vi "Plot_Channels.vi"() -> (5 "Plug in titles":string[](array[string]), 7 "Plug in values":string[](array[string]))   [LabVIEW 2011]
uses:
  Globals/Meas_global.vi
panel:
  out "Stats out":T1
  out "Size 2":i32
  out "Size 1":i32
  out "Size 0":i32
  in  "interp. method":i32(ring) items=["nearest", "linear", "spline", "cubic Hermite", "Lagrange"]
  in  "index 2":i32=3
  out "XY Graph":cluster{"Time (ms)":dbl[], "Eng Values":dbl[]}[](graph)
  in  "index 1":i32=1
  in  "index 0":i32
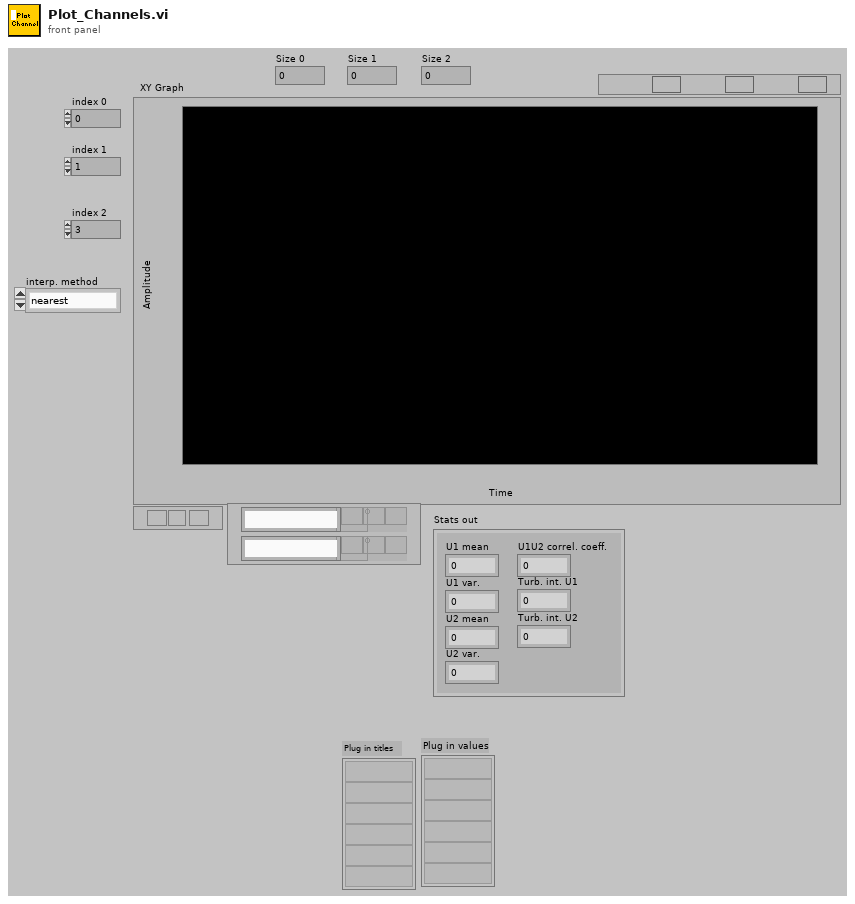
[diagram p1: front panel]
types:
  T1 = cluster{"U1 mean":dbl, "U1 var.":dbl, "U2 mean":dbl, "U2 var.":dbl, "U1U2 correl. coeff.":dbl, "Turb. int. U1":dbl, "Turb. int. U2":dbl}
  T2 = typedef "Analysis_info_cluster.ctl" = cluster{"Colour":u32, "Inst type":T3, "Inst name":string, "Symbol":string, "Code name":string, "Extra Info":string, "Inst Array":T4, "Index":i32, "Voltage Index":i32, "Extra Titles":string[], "Extra Values":string[], "Eng Values":dbl[], "Time (ms)":dbl[], "TT / Voltage":dbl[], "U":dbl, "u^2":dbl, "u^3":dbl, "u^4":dbl, "Skew_u":dbl, "Kurt_u":dbl, "Mean % Err":dbl, "% u'/U":dbl}
  T3 = typedef "Inst_type.ctl" = enum16{"Propeller anemometer", "Raw voltage", "Pressure Transducer", "Pitot-static tube", "Preston tube", "Hot wire", "Cross wire 1", "Cross wire 2", "Generic Linear", "Generic Polynomial", "Generic BackPoly", "Fast FID", "Thermocouple", "Cold wire", "Pulsed Wire", "LDA Vel", "LDA Tran time", "LDA Arr time"}
  T4 = typedef "Instrument_Array.ctl" = enum16{"PWA", "LDA", "Analogue"}
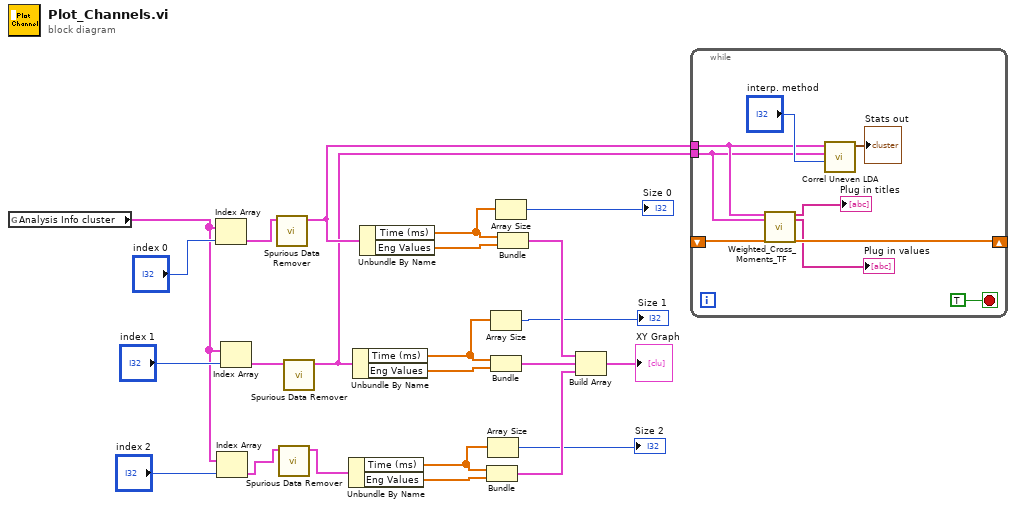
[diagram p0: block diagram]
diagram:
  n1 = global read "Meas_global.vi" "Analysis Info cluster"() -> (w7:T2[])
  n2 = Index Array(array=w7, index="index 0") -> (element=w6:T2)
  n3 = Index Array(array=w7, index="index 2") -> (element=w4:T2)
  n4 = Index Array(array=w7, index="index 1") -> (element=w2:T2)
  n5 = call "Spurious Data Remover.vi"("Cluster 1"=w6) -> ("Cluster 1 Spurious points removed"=w5:T2)  [unwired: 10 in]
  n6 = call "Spurious Data Remover.vi"("Cluster 1"=w4) -> ("Cluster 1 Spurious points removed"=w3:T2)  [unwired: 10 in]
  n7 = call "Spurious Data Remover.vi"("Cluster 1"=w2) -> ("Cluster 1 Spurious points removed"=w1:T2)  [unwired: 10 in]
  n8 = Unbundle By Name(w3) -> ("Time (ms)"=w11:dbl[], "Eng Values"=w16:dbl[])
  n9 = Unbundle By Name(w1) -> ("Time (ms)"=w12:dbl[], "Eng Values"=w20:dbl[])
  n10 = Unbundle By Name(w5) -> ("Time (ms)"=w13:dbl[], "Eng Values"=w21:dbl[])
  n11 = Bundle("Time (ms)"=w11, "Eng Values"=w16) -> (w14:cluster{"Time (ms)":dbl[], "Eng Values":dbl[]})  [unwired: 1 in]
  n12 = Array Size(array=w11) -> (size(s)=→"Size 2":i32)
  n13 = Array Size(array=w12) -> (size(s)=→"Size 1":i32)
  n14 = Bundle("Time (ms)"=w12, "Eng Values"=w20) -> (w19:cluster{"Time (ms)":dbl[], "Eng Values":dbl[]})  [unwired: 1 in]
  n15 = Array Size(array=w13) -> (size(s)=→"Size 0":i32)
  n16 = Bundle("Time (ms)"=w13, "Eng Values"=w21) -> (w18:cluster{"Time (ms)":dbl[], "Eng Values":dbl[]})  [unwired: 1 in]
  n17 = Build Array(w18, w19, w14) -> (→"XY Graph":cluster{"Time (ms)":dbl[], "Eng Values":dbl[]}[])
  n18 = while {
    tunnel: w5 -> [w30]
    tunnel: w1 -> [w29]
    shift-right: [w27] -> _
    shift-left: _ -> [w26]
    stop <- TRUE stop-if-true
    n19 = call "Weighted_Cross_Moments_TF.vi"("Cluster 1"=w30, "Cluster 2"=w29, "Shift in"=w26) -> ("Headers"=→"Plug in titles":string[], "Results"=→"Plug in values":string[], "Shift out"=w27:dbl[])  [unwired: 14 in]
    n20 = call "Correl Uneven LDA.vi"("interp. method"="interp. method", "Cluster 2"=w29, "Cluster 1"=w30) -> ("Stats out"=→"Stats out":T1)  [unwired: 8 in]
  }
